vi "Normal Distribution.vi"(1 "x":dbl format="%0.4f") -> (0 "probability":dbl format="%0.4f")   [LabVIEW 2017, in "NI_AALPro.lvlib"]
doc: "LabVIEW no longer supports this VI. Use the Continuous CDF VI (Normal instance) instead. Computes the one-sided <B>probability</B>, p, of the normally distributed random variable, <B>x</B>. The Normal Distribution VI computes the one-sided <B>probability</B> of <B>x</B> such that the following condition is satisfied: p = Prob {X <= <B>x</B>}, where X is standard Normally distributed, p is the <B>probability</B>, and <B>x</B> is the value. The Normal Distribution VI computes only the one-sided probability. You can obtain the two-sided probability, (p = Prob {-x <= X <= x}), using the following equation: p1 = 1 - 2(1 - p) = 2p - 1 = 2Prob{X <= x} - 1."
uses:
  NI_AALPro.lvlib
  <resource>/lvanlys.dll
panel:
  # "Normal Distribution"
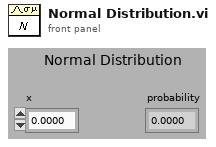
[diagram p1: front panel]
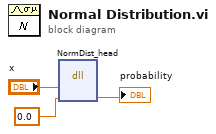
[diagram p0: block diagram]
diagram:
  n1 = dll-call lib="C:/Program Files (x86)/National Instruments/LabVIEW 2017/resource/lvanlys.*" fn="NormDist_head"("x"="x", 0.0) -> (→"probability":dbl)  [unwired: 5 in, 2 out]
